vi "sc5511a_set_rf_mode.vi"(0 "deviceHandle":u32 format="%.0x", 2 "RF Mode":u8(ring) items=["Fixed", "List/Sweep"], 5 "error in":errorcluster) -> (14 "deviceHandle":u32 format="%.0x", 19 "error out":errorcluster)   [LabVIEW 2010]
uses:
  sc5511a_rs232.dll
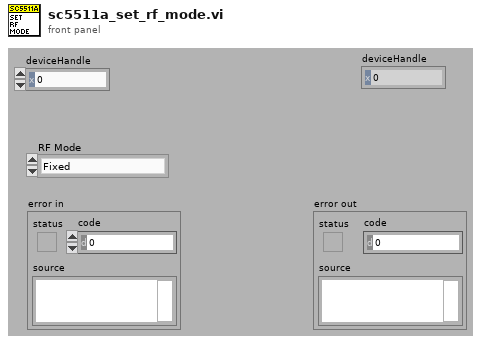
[diagram p1: front panel]
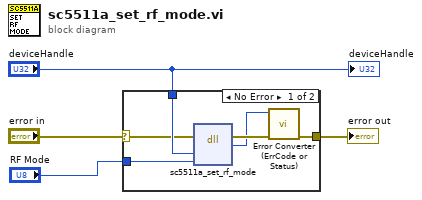
[diagram p0: block diagram]
diagram:
  n1 = case shown="No Error" "error in" {
    selector: "error in" -> [w5 w11]
    tunnel: [w10 w11] -> w4
    tunnel: "deviceHandle" -> [w7 _]
    tunnel: "RF Mode" -> [w6 _]
    frame No Error {
      n2 = dll-call lib="sc5511a_rs232.dll" fn="sc5511a_set_rf_mode"(error in=w5, "deviceHandle"=w7, "rf_mode"=w6) -> (error out=w9:errorcluster, "return type"=w8:i32)  [unwired: 4 in, 1 out]
      n3 = call "Error Converter (ErrCode or Status).vi"("error in (no error)"=w9, "error code"=w8) -> ("error out"=w10:errorcluster)  [unwired: 9 in]
    }
    frame Error {
    }
  }
  "error out" <- w4
  "deviceHandle" <- "deviceHandle"
